vi "Transfer Count (Transfer Group).vi"(8 "error in (no error)":errorcluster, 11 "Transfer Group Configuration in":T1 {"Transfers"."channels"."string offset" format="%d bytes"}) -> (0 "error out":errorcluster, 2 "transfer count":i32, 3 "Transfer Group Configuration out":T1 {"Transfers"."channels"."string offset" format="%d bytes"})   [LabVIEW 2017, in "DSF Core.lvlib"]
uses:
  Typedefs/DSF Engine Transfer Group Configuration.ctl
  Typedefs/DSF Direction.ctl
  Typedefs/DSF Timing Info.ctl
  Typedefs/DSF Settings Info.ctl
  Typedefs/DSF Engine Transfer Configuration.ctl
  Typedefs/DSF Byte Order.ctl
  Typedefs/DSF Engine Channel Configuration.ctl
  Typedefs/DSF Data Type.ctl
  DSF Core.lvlib
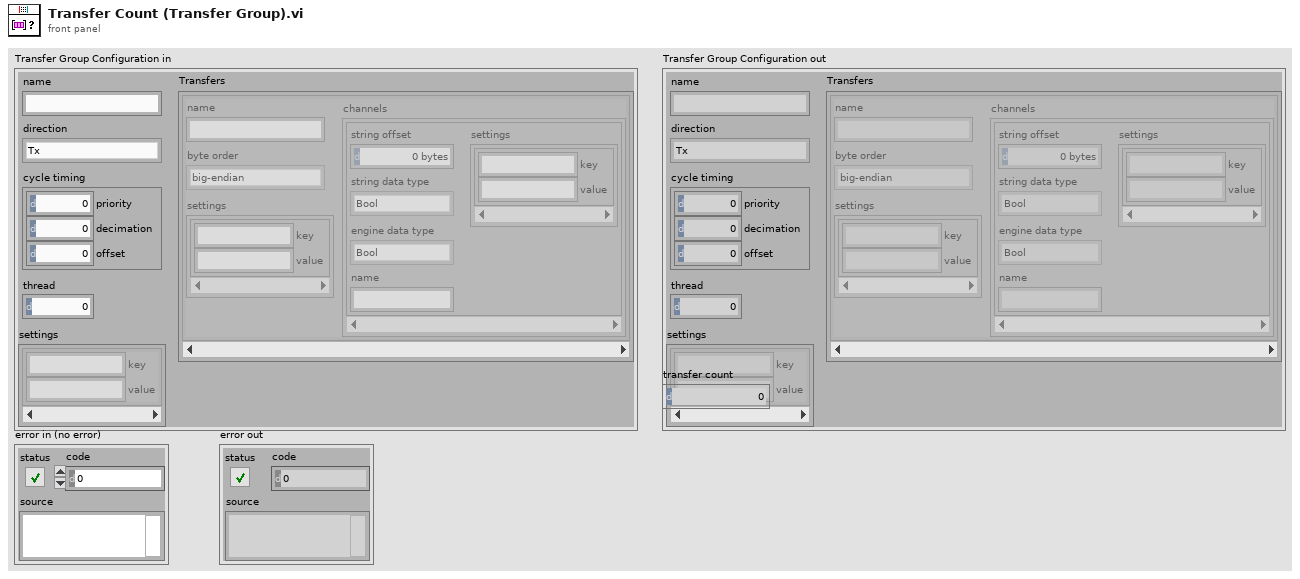
[diagram p1: front panel]
types:
  T1 = typedef "DSF Core.lvlib/DSF Engine Transfer Group Configuration.ctl" = cluster{"name":string, "direction":T2, "cycle timing":T3, "thread":i32, "settings":T4, "Transfers":T5[]}
  T2 = typedef "DSF Core.lvlib/DSF Direction.ctl" = enum8{"Tx", "Rx"}
  T3 = typedef "DSF Core.lvlib/DSF Timing Info.ctl" = cluster{"priority":u64, "decimation":u64, "offset":u64}
  T4 = typedef "DSF Core.lvlib/DSF Settings Info.ctl" = cluster{"key":string, "value":string}[]
  T5 = typedef "DSF Core.lvlib/DSF Engine Transfer Configuration.ctl" = cluster{"name":string, "byte order":T6, "settings":T4, "channels":T7[]}
  T6 = typedef "DSF Core.lvlib/DSF Byte Order.ctl" = enum8{"big-endian", "little-endian"}
  T7 = typedef "DSF Core.lvlib/DSF Engine Channel Configuration.ctl" = cluster{"string offset":u64, "string data type":T8, "engine data type":T8, "name":string, "settings":T4}
  T8 = typedef "DSF Core.lvlib/DSF Data Type.ctl" = enum8{"Bool", "SGL", "DBL", "I8", "I16", "I32", "I64", "U8", "U16", "U32", "U64"}
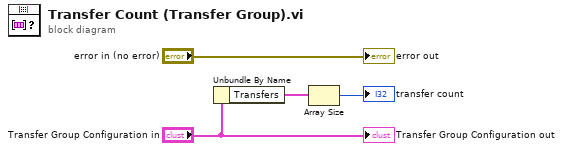
[diagram p0: block diagram]
diagram:
  n1 = Unbundle By Name("Transfer Group Configuration in") -> ("Transfers"=w2:T5[])
  n2 = Array Size(array=w2) -> (size(s)=→"transfer count":i32)
  "Transfer Group Configuration out" <- "Transfer Group Configuration in"
  "error out" <- "error in (no error)"
